vi "mutil channel.vi"() -> ()   [LabVIEW 2022 SP3]
uses:
  <vilib>/express/express analysis/Spectral/XNode/ExpressSpectralMeasurementsBlockNode.xnode
  <vilib>/express/express analysis/Spectral/Block/exnSpectralBlock spectral measurements power poly.vi
  <vilib>/express/express analysis/Spectral/Block/exnSpectralBlock spectral measurements power DDT.vi
panel:
  out "Baseband 2":dynamicdata(graph)
  in  "WAV Sample Rate 2":dbl=44100.0 caption="dt"
  in  "LPF Cut-Off 2":dbl=10000.0 caption="Lower Cut-Off"
  out "Comparision 2":dynamicdata(graph)
  in  "DC Offset 2":dbl=1.0
  in  "Carrier Amp. 2":dbl=1.0 caption="Amplitude"
  in  "Modulation Index 2":dbl(slide)=1.0 scale=0.0..5.0
  in  "Carrier Freq. 2":dbl=100000.0 caption="Frequency"
  in  "Mod. Freq. 2":dbl=2000.0 caption="Frequency"
  in  "WAV Sample Rate":dbl=44100.0 caption="dt"
  in  "Mod. Freq.":dbl=2000.0 caption="Frequency"
  in  "LPF Cut-Off":dbl=10000.0 caption="Lower Cut-Off"
  in  "AWGN (dB)":dbl(slide)=0.6 caption="Standard deviation" scale=-20.0..30.0
  out "Comparision":dynamicdata(graph)
  out "Baseband":dynamicdata(graph)
  out "AM FFT":dynamicdata(graph)
  out "AM Wave":dynamicdata(graph)
  in  "DC Offset":dbl=1.0
  in  "Carrier Amp.":dbl=1.0 caption="Amplitude"
  in  "stop":bool
  in  "Modulation Index":dbl(slide)=1.0 scale=0.0..5.0
  in  "Carrier Freq.":dbl=100000.0 caption="Frequency"
  out "After Rectifier":dynamicdata(graph)=[{"t0"=timestamp(0 s since 1904-01-01), "dt"=10.0, "Y"=array[50000 elements], "attributes"=variant("NI_ChannelName"=variant(string "Sine (Power Spectrum)"), "NI_ExpIsRelativeTime"=variant(bool TRUE), "NI_ExpStartTimeStamp"=variant(timestamp timestamp(3635665779.2842293 s since 1904-01-01)), "NI_ExpTimeStamp"=variant(timestamp timestamp(3635665779.2842293 s since 1904-01-01)), "NI_ExpXDimension"=variant(string "f"), "NI_OriginalChannelName"=variant(string "Sine"))}]
  # "Amplitude Modulation"
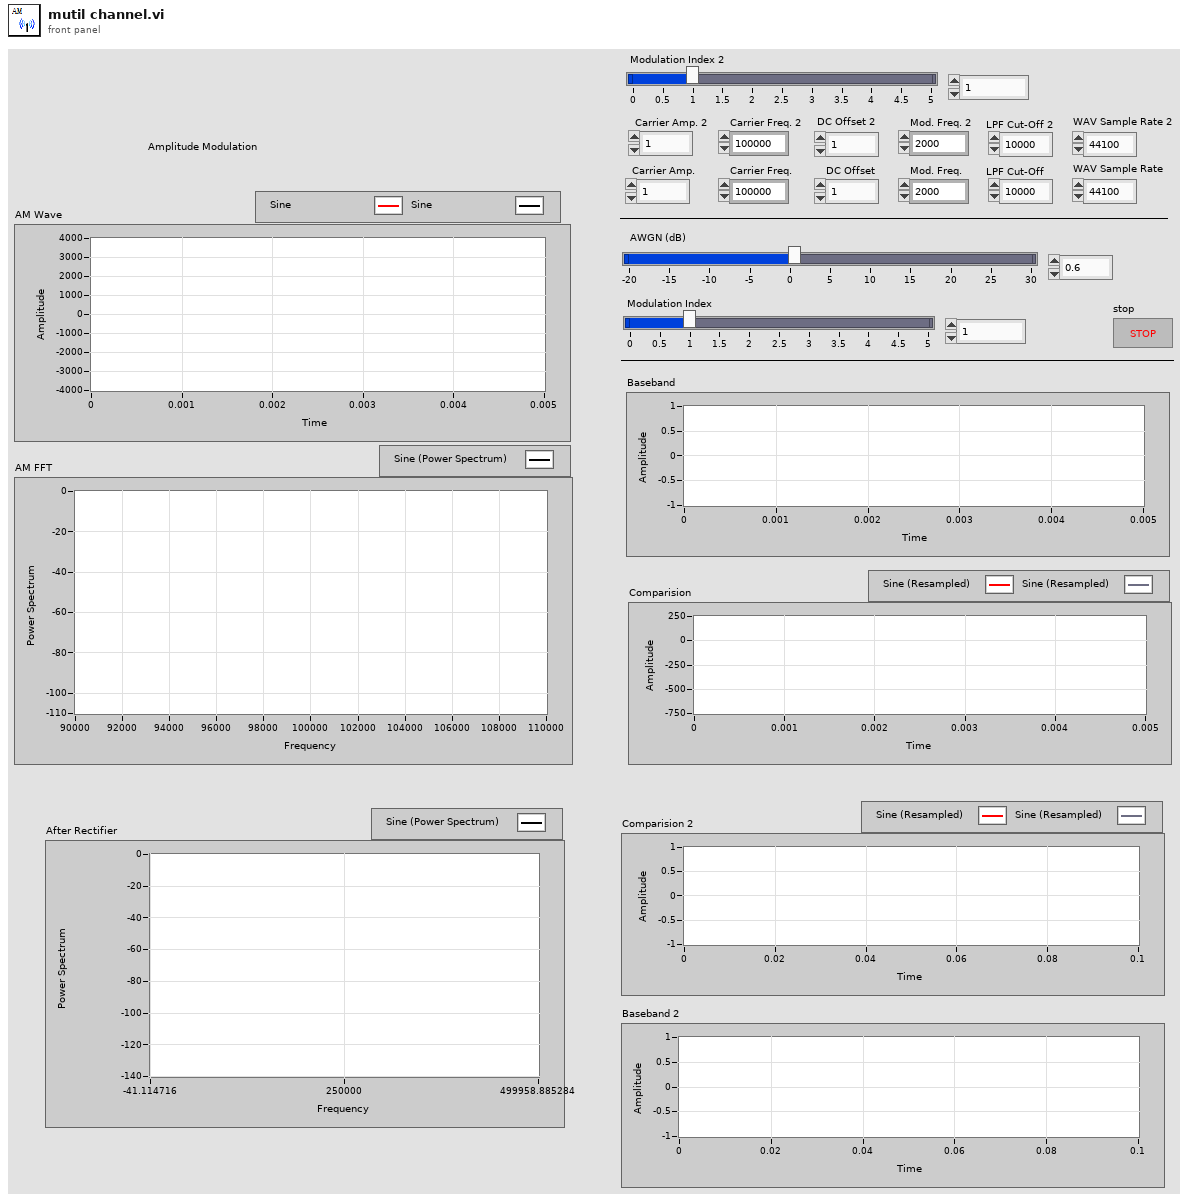
[diagram p1: front panel]
types:
  T1 = cluster{"averaging mode":u16, "weighting mode":u16, "number of averages":u32}
  T2 = cluster{"dB On (F)":bool, "unwrap phase (F)":bool, "convert to degree (F)":bool}
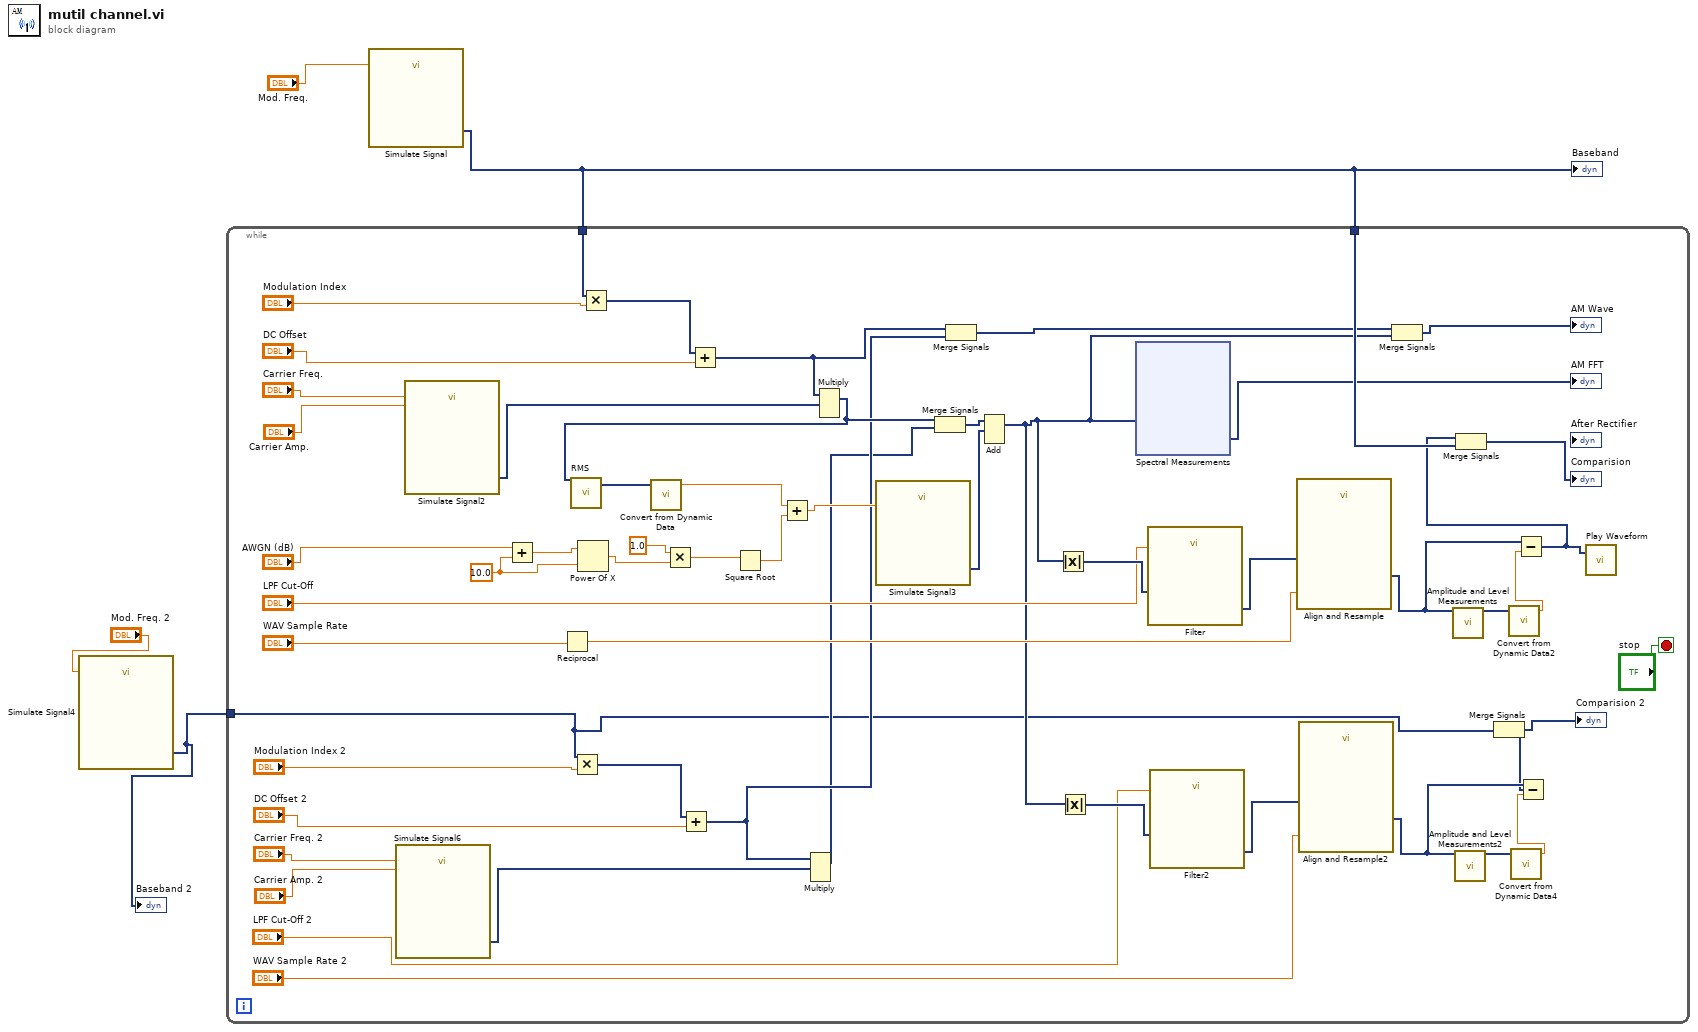
[diagram p0: block diagram]
diagram:
  n1 = call "Simulate Signal4"("Frequency"="Mod. Freq. 2") -> ("Sine"=w1:dynamicdata)  [unwired: 13 in, 1 out]
  "Baseband 2" <- w1
  n2 = call "Simulate Signal"("Frequency"="Mod. Freq.") -> ("Sine"=w3:dynamicdata)  [unwired: 13 in, 1 out]
  "Baseband" <- w3
  n3 = while {
    tunnel: w3 -> [w55]
    tunnel: w3 -> [w29]
    tunnel: w1 -> [w8]
    stop <- "stop" stop-if-true
    w49 = 10.0
    n4 = call "Simulate Signal6"("Frequency"="Carrier Freq. 2", "Amplitude"="Carrier Amp. 2") -> ("Sine"=w20:dynamicdata)  [unwired: 12 in, 1 out]
    n5 = call "Simulate Signal2"("Frequency"="Carrier Freq.", "Amplitude"="Carrier Amp.") -> ("Sine"=w52:dynamicdata)  [unwired: 12 in, 1 out]
    n6 = Add(x="AWGN (dB)", y=w49) -> (x+y=w50:dbl)
    n7 = Reciprocal(x="WAV Sample Rate") -> (1/x=w36:dbl)
    n8 = Multiply(x=w8, y="Modulation Index 2") -> (x*y=w24:dynamicdata)
    n9 = Power Of X(1:w49, 2:w50) -> (0:w48:dbl)
    n10 = Multiply(x=w55, y="Modulation Index") -> (x*y=w57:dynamicdata)
    n11 = Multiply(x=1.0, y=w48) -> (x*y=w46:dbl)
    n12 = Add(x=w24, y="DC Offset 2") -> (x+y=w13:dynamicdata)
    n13 = Add(x=w57, y="DC Offset") -> (x+y=w35:dynamicdata)
    n14 = Square Root(x=w46) -> (sqrt(x)=w45:dbl)
    n15 = Multiply(1:w20, 2:w13) -> (0:w11:dynamicdata)  [unwired: 1 in, 1 out]
    n16 = Multiply(1:w52, 2:w35) -> (0:w41:dynamicdata)  [unwired: 1 in, 1 out]
    n17 = call "RMS"("Signals"=w41) -> ("RMS"=w26:dynamicdata)  [unwired: 12 in, 2 out]
    n18 = call "Convert from Dynamic Data"("Dynamic Data Type"=w26) -> ("Scalar"=w42:dbl)  [unwired: 3 in]
    n19 = Add(x=w42, y=w45) -> (x+y=w44:dbl)
    n20 = call "Simulate Signal3"("Standard deviation"=w44) -> ("DC with Gaussian Noise"=w43:dynamicdata)  [unwired: 13 in, 1 out]
    n21 = Merge Signals(w41, w11) -> (w12:dynamicdata)
    n22 = Merge Signals(w35, w13) -> (w14:dynamicdata)
    n23 = Add(1:w43, 2:w12) -> (0:w10:dynamicdata)  [unwired: 1 in, 1 out]
    n24 = Absolute Value(x=w10) -> (abs(x)=w40:dynamicdata)
    n25 = Absolute Value(x=w10) -> (abs(x)=w19:dynamicdata)
    n26 = xnode "Spectral Measurements"("Signals"=w10) -> ("Power Spectrum"=→"AM FFT":dynamicdata)  [unwired: 1 in, 1 out]
    n27 = call "Filter"("Lower Cut-Off"="LPF Cut-Off", "Signal"=w40) -> ("Filtered Signal"=w38:dynamicdata)  [unwired: 8 in, 1 out]
    n28 = call "Filter2"("Lower Cut-Off"="LPF Cut-Off 2", "Signal"=w19) -> ("Filtered Signal"=w18:dynamicdata)  [unwired: 8 in, 1 out]
    n29 = call "Align and Resample"("dt"=w36, "Signals"=w38) -> ("Resampled Signals"=w31:dynamicdata)  [unwired: 7 in, 2 out]
    n30 = call "Align and Resample2"("dt"="WAV Sample Rate 2", "Signals"=w18) -> ("Resampled Signals"=w15:dynamicdata)  [unwired: 7 in, 2 out]
    n31 = Merge Signals(w14, w10) -> (→"AM Wave":dynamicdata)
    n32 = call "Amplitude and Level Measurements"("Signals"=w31) -> ("Mean (DC)"=w33:dynamicdata)  [unwired: 13 in, 1 out]
    n33 = call "Amplitude and Level Measurements2"("Signals"=w15) -> ("Mean (DC)"=w17:dynamicdata)  [unwired: 13 in, 1 out]
    n34 = call "Convert from Dynamic Data2"("Dynamic Data Type"=w33) -> ("Scalar"=w32:dbl)  [unwired: 3 in]
    n35 = call "Convert from Dynamic Data4"("Dynamic Data Type"=w17) -> ("Scalar"=w16:dbl)  [unwired: 3 in]
    n36 = Subtract(x=w31, y=w32) -> (x-y=w28:dynamicdata)
    n37 = Merge Signals(w28, w29) -> (→"Comparision":dynamicdata)
    n38 = Subtract(x=w15, y=w16) -> (x-y=w5:dynamicdata)
    n39 = Merge Signals(w5, w8) -> (→"Comparision 2":dynamicdata)
    n40 = call "Play Waveform"("Data"=w28) -> ()  [unwired: 18 in, 1 out]
  }
